vi "显示PCB序号.vi"(7 "Font, Size & Style":T4={"Desired Font (Application)"=enum."User-specified Font", "[User-specified Font]"={"Font Name"="", "Size"=40, "Strikeout?"=FALSE, "Italic?"=FALSE, "Underline?"=FALSE, "Outline?"=FALSE, "Shadow?"=FALSE, "Bold?"=TRUE, "Rotation Angle"=0.0}, "Horizontal Alignment"=0, "Vertical Alignment"=0} {"Horizontal Alignment" items=["Left", "Center", "Right"]; "Vertical Alignment" items=["Bottom", "Top", "Baseline"]}, 8 "显示坐标":cluster{dbl, "Numeric":dbl}[](array[cluster]), 9 "ModelEditInfo":T1={"Root"=path "", "AllModelFold"=path "", "AllModelNamePath"=path "", "所有零件型号"=[], "当前零件型号"="", "所有建立零件信息"=[], "当前零件序号"=0, "当前产品所有点位信息"={"当前点位序号"=0, "点位信息路径"=path "", "CAD点位坐标路径"=path "", "点位信息表"=[], "CAD图纸点位个数"=0}, "当前产品信息"={"产品型号"="", "载具上放几片PCB"=0, "1片PCB锁几颗螺丝"=0, "CAD点位坐标文档路径"=path "", "托盘1螺丝锁紧程式序号"=0, "托盘2螺丝锁紧程式序号"=0, "托盘3螺丝锁紧程式序号"=0, "托盘4螺丝锁紧程式序号"=0, "托盘5螺丝锁紧程式序号"=0, "托盘6螺丝锁紧程式序号"=0, "托盘7螺丝锁紧程式序号"=0, "托盘8螺丝锁紧程式序号"=0, "预锁程式序号"=0, "复锁程式序号"=0, "复锁拍照点与Mark拍照点高度差"=1.0, "取料点与P2高度差"=1.0, "拍PCB孔曝光时间"=0, "取料拍螺帽曝光时间"=0, "复锁拍螺帽曝光时间"=0, "下相机曝光时间"=0}, "所有螺丝和垫片型号Path"=path "", "8个供料盘是否供料-1PCB(去除未勾选的)"=[], "8个供料盘是否拍照取料"=[], "自动锁螺丝: 1PCB每颗螺丝来自哪个供料盘U8(去除未勾选的)"=[], "自动锁螺丝: 1PCB每颗螺丝拧紧程式编号U8(去除未勾选的)"=[], "4个预锁程式+4个复锁程式编号U8"=[], "自动锁螺丝: 锁螺丝相对拍照时旋转角度-多片PCB(去除未勾选的)"=[], "1PCB上自动锁螺丝个数(去除未勾选的)"=0, "自动锁螺丝: 放料点相对拍照点高度差-多片PCB(去除未勾选的)"=[], "8个供料盘是否供料(包括未勾选的)"=[], "已勾选的自动锁螺丝点位供料盘设定错误"=FALSE, "自动锁螺丝: 1PCB每颗螺丝外径*10(去除未勾选的)"=[], "拧紧程式参数"={"所有拧紧程式参数表路径"=path "", "所有拧紧程式参数表"=[], "所有拧紧程式参数表当前行"=0}, "已勾选的自动锁螺丝点位拧紧程式序号设定错误"=FALSE} {"当前产品信息"."载具上放几片PCB" min=1 max=4; "当前产品信息"."托盘8螺丝锁紧程式序号" min=1 max=150 step=1; "当前产品信息"."托盘7螺丝锁紧程式序号" min=1 max=150 step=1; "当前产品信息"."托盘6螺丝锁紧程式序号" min=1 max=150 step=1; "当前产品信息"."托盘5螺丝锁紧程式序号" min=1 max=150 step=1; "当前产品信息"."复锁程式序号" min=1 max=150 step=1; "当前产品信息"."预锁程式序号" min=1 max=150 step=1; "当前产品信息"."托盘4螺丝锁紧程式序号" min=1 max=150 step=1; "当前产品信息"."托盘3螺丝锁紧程式序号" min=1 max=150 step=1; "当前产品信息"."托盘2螺丝锁紧程式序号" min=1 max=150 step=1; "当前产品信息"."托盘1螺丝锁紧程式序号" min=1 max=150 step=1}, 11 "Img输入":T3) -> (3 "Img输出":T3)   [LabVIEW 2014]
uses:
  <vilib>/vision/Image Controls.llb/IMAQ Image.ctl
  ModelEditSubVIs/ModeEditeControl.ctl
  ModelEditSubVIs/ModelInfo.ctl
panel:
  out "数组":cluster{dbl, dbl}[](array[cluster])
  # "mm"
  # "mm"
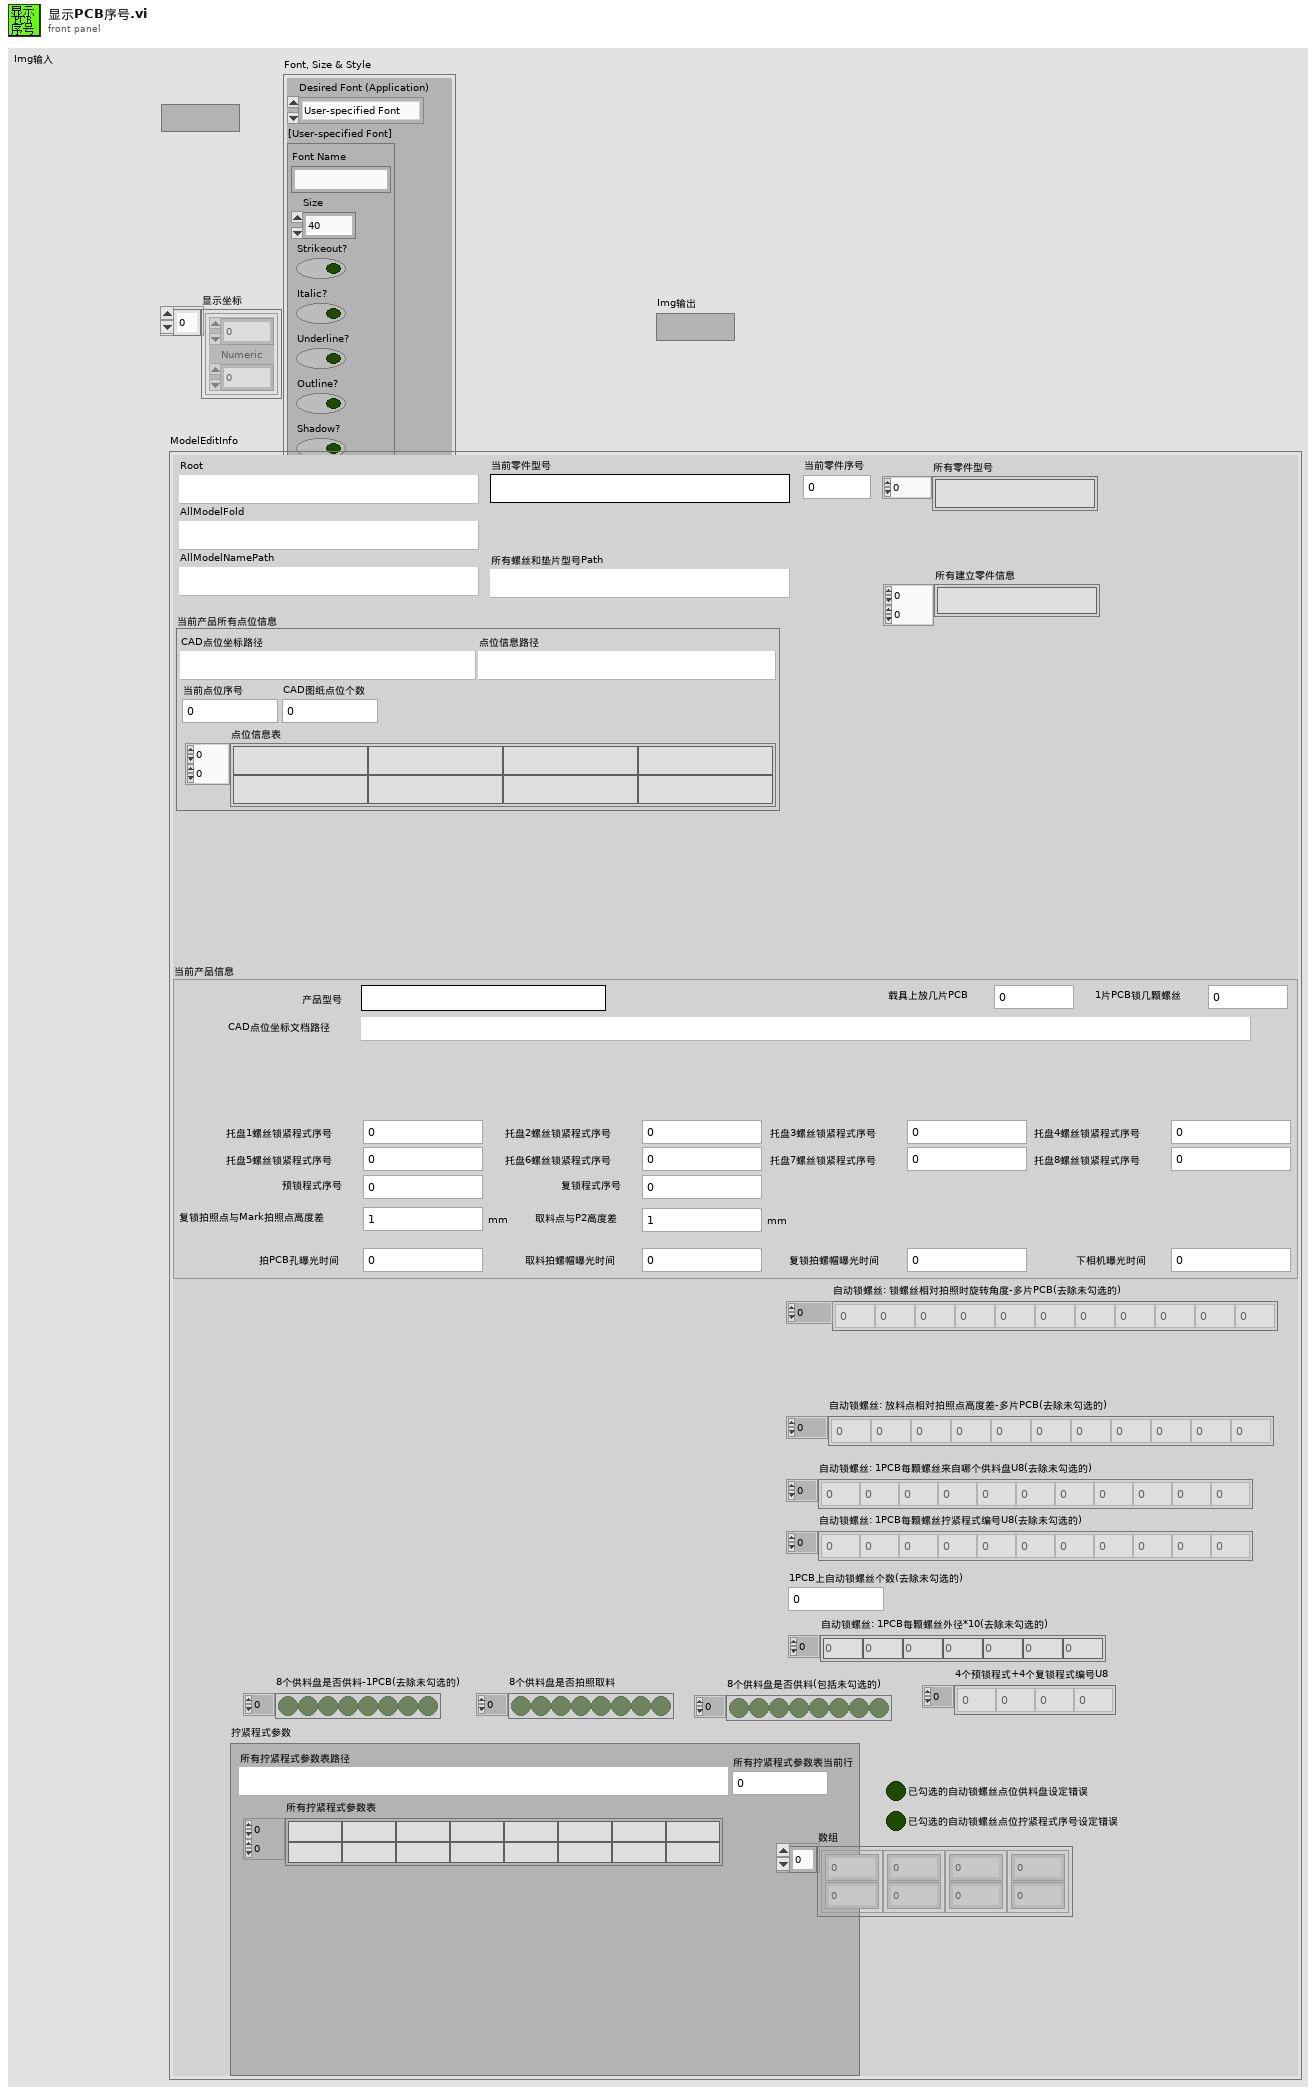
[diagram p1: front panel]
types:
  T1 = typedef "ModeEditeControl.ctl" = cluster{"Root":path, "AllModelFold":path, "AllModelNamePath":path, "所有零件型号":string[], "当前零件型号":string, "所有建立零件信息":string[][], "当前零件序号":i32, "当前产品所有点位信息":cluster{"当前点位序号":i32, "点位信息路径":path, "CAD点位坐标路径":path, "点位信息表":string[][], "CAD图纸点位个数":i32}, "当前产品信息":T2, "所有螺丝和垫片型号Path":path, "8个供料盘是否供料-1PCB(去除未勾选的)":bool[], "8个供料盘是否拍照取料":bool[], "自动锁螺丝: 1PCB每颗螺丝来自哪个供料盘U8(去除未勾选的)":u8[], "自动锁螺丝: 1PCB每颗螺丝拧紧程式编号U8(去除未勾选的)":u8[], "4个预锁程式+4个复锁程式编号U8":u8[], "自动锁螺丝: 锁螺丝相对拍照时旋转角度-多片PCB(去除未勾选的)":i32[], "1PCB上自动锁螺丝个数(去除未勾选的)":i32, "自动锁螺丝: 放料点相对拍照点高度差-多片PCB(去除未勾选的)":dbl[], "8个供料盘是否供料(包括未勾选的)":bool[], "已勾选的自动锁螺丝点位供料盘设定错误":bool, "自动锁螺丝: 1PCB每颗螺丝外径*10(去除未勾选的)":u32[], "拧紧程式参数":cluster{"所有拧紧程式参数表路径":path, "所有拧紧程式参数表":string[][], "所有拧紧程式参数表当前行":i32}, "已勾选的自动锁螺丝点位拧紧程式序号设定错误":bool}
  T2 = typedef "ModelInfo.ctl" = cluster{"产品型号":string, "载具上放几片PCB":u16, "1片PCB锁几颗螺丝":u16, "CAD点位坐标文档路径":path, "托盘1螺丝锁紧程式序号":u32, "托盘2螺丝锁紧程式序号":u32, "托盘3螺丝锁紧程式序号":u32, "托盘4螺丝锁紧程式序号":u32, "托盘5螺丝锁紧程式序号":u32, "托盘6螺丝锁紧程式序号":u32, "托盘7螺丝锁紧程式序号":u32, "托盘8螺丝锁紧程式序号":u32, "预锁程式序号":u32, "复锁程式序号":u32, "复锁拍照点与Mark拍照点高度差":dbl, "取料点与P2高度差":dbl, "拍PCB孔曝光时间":u32, "取料拍螺帽曝光时间":u32, "复锁拍螺帽曝光时间":u32, "下相机曝光时间":u32}
  T3 = typedef "IMAQ Image.ctl" = refnum<image>
  T4 = cluster{"Desired Font (Application)":enum16{"User-specified Font", "Application Font", "System Font", "Dialog Font"}, "[User-specified Font]":cluster{"Font Name":string, "Size":i16, "Strikeout?":bool, "Italic?":bool, "Underline?":bool, "Outline?":bool, "Shadow?":bool, "Bold?":bool, "Rotation Angle":dbl}, "Horizontal Alignment":i16, "Vertical Alignment":i16}
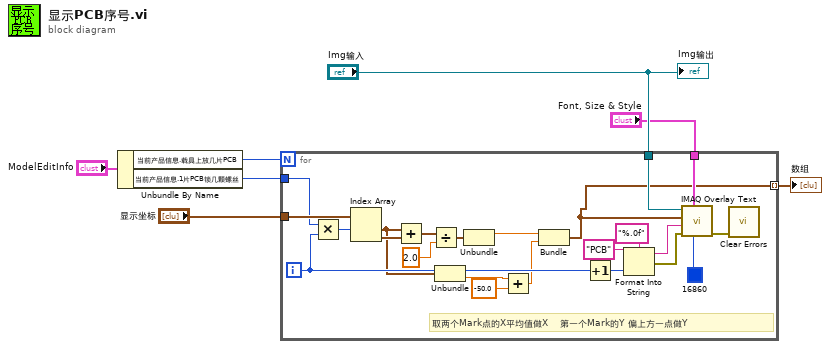
[diagram p0: block diagram]
diagram:
  n1 = Unbundle By Name("ModelEditInfo") -> ("当前产品信息.载具上放几片PCB"=w3:u16, "当前产品信息.1片PCB锁几颗螺丝"=w2:u16)
  n2 = for {
    N: w3 -> [_]
    tunnel: "Img输入" -> [w30]
    tunnel: "显示坐标" -> [w22]
    tunnel: "Font, Size & Style" -> [w29]
    tunnel: w2 -> [w21]
    tunnel: [w9] -> w1 mode=indexing
    i -> [w20]
    # "取两个Mark点的X平均值做X    第一个Mark的Y 偏上方一点做Y"
    n3 = Multiply(x=w21, y=w20) -> (x*y=w19:i32)
    n4 = Index Array(array=w22, index #1=w19) -> (element #1=w15:cluster{dbl, "Numeric":dbl}, element #2=w18:cluster{dbl, "Numeric":dbl})  [unwired: 1 in]
    n5 = Add(x=w15, y=w18) -> (x+y=w17:cluster{dbl, "Numeric":dbl})
    n6 = Divide(x=w17, y=2.0) -> (x/y=w14:cluster{dbl, "Numeric":dbl})
    n7 = Unbundle(w15) -> ("Numeric"=w8:dbl)  [unwired: 1 out]
    n8 = Unbundle(w14) -> (w12:dbl)  [unwired: 1 out]
    n9 = Add(x=w8, y=-50.0) -> (x+y=w11:dbl)
    n10 = Bundle(w12, w11) -> (w9:cluster{dbl, dbl})  [unwired: 1 in]
    n11 = Increment(x=w20) -> (x+1=w23:i32)
    n12 = Format Into String(format string="%.0f" ("格式字符串"), initial string="PCB" ("初始字符串"), w23) -> (resulting string=w28:string, error out=w26:errorcluster)  [unwired: 1 in]
    n13 = call "IMAQ Overlay Text"("Text Color (black)"=u32 16860, "Font, Size & Style"=w29, "error in (no error)"=w26, "String"=w28, "Origin"=w9, "Image"=w30) -> ("error out"=w25:errorcluster)  [unwired: 4 in, 1 out]
    n14 = call <vilib>:"Clear Errors.vi"("error in (no error)"=w25) -> ()  [unwired: 5 in, 2 out]
  }
  "数组" <- w1
  "Img输出" <- "Img输入"
